vi "Is Element Owned.vi"(10 "Nested Object":refnum<vi>, 11 "Relative Object":refnum<vi>) -> (3 "is owned?":bool)   [LabVIEW 2014]
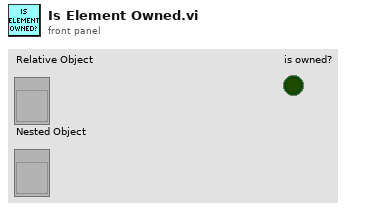
[diagram p1: front panel]
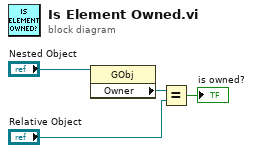
[diagram p0: block diagram]
diagram:
  n1 = property class="GObj"(reference="Nested Object") -> ("Owner"=w2:refnum<vi>)  [unwired: 1 in, 2 out]
  n2 = Equal?(x=w2, y="Relative Object") -> (x = y?=→"is owned?":bool)
